vi "多从板对应参数.vi"(2 "从板个数":dbl=1.0) -> (0 "输出数组":string[](array[string]))   [LabVIEW 2013]
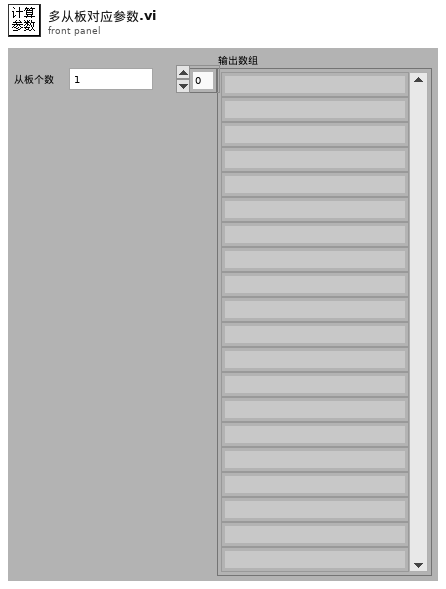
[diagram p1: front panel]
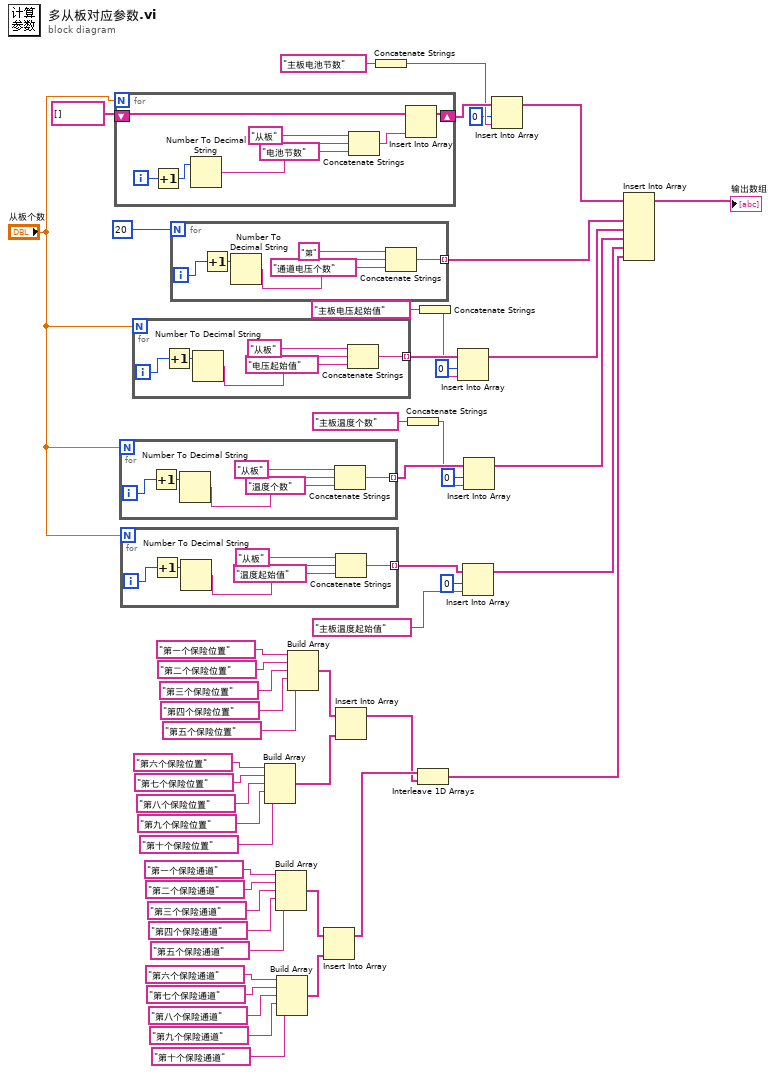
[diagram p0: block diagram]
diagram:
  n1 = for {
    N: "从板个数" -> [_]
    shift-right: [w56] -> w45
    shift-left: string[] [] -> [w55]
    i -> [w54]
    n2 = Increment(x=w54) -> (x+1=w52:i32)
    n3 = Number To Decimal String(number=w52) -> (decimal integer string=w58:string)  [unwired: 1 out]
    n4 = Concatenate Strings("从板" ("字符串"), w58, "电池节数" ("字符串")) -> (w53:string)
    n5 = Insert Into Array(array=w55, new element=w53) -> (w56:string[])  [unwired: 1 in]
  }
  n6 = for {
    N: "从板个数" -> [_]
    tunnel: [w60] -> w41 mode=indexing
    i -> [w65]
    n7 = Increment(x=w65) -> (x+1=w64:i32)
    n8 = Number To Decimal String(number=w64) -> (decimal integer string=w62:string)  [unwired: 1 out]
    n9 = Concatenate Strings("从板" ("字符串"), w62, "温度个数" ("字符串")) -> (w60:string)
  }
  n10 = for {
    N: "从板个数" -> [_]
    tunnel: [w66] -> w30 mode=indexing
    i -> [w71]
    n11 = Increment(x=w71) -> (x+1=w70:i32)
    n12 = Number To Decimal String(number=w70) -> (decimal integer string=w68:string)  [unwired: 1 out]
    n13 = Concatenate Strings("从板" ("字符串"), w68, "温度起始值" ("字符串")) -> (w66:string)
  }
  n14 = for {
    N: "从板个数" -> [_]
    tunnel: [w72] -> w37 mode=indexing
    i -> [w77]
    n15 = Increment(x=w77) -> (x+1=w76:i32)
    n16 = Number To Decimal String(number=w76) -> (decimal integer string=w74:string)  [unwired: 1 out]
    n17 = Concatenate Strings("从板" ("字符串"), w74, "电压起始值" ("字符串")) -> (w72:string)
  }
  n18 = for {
    N: 20 -> [_]
    tunnel: [w78] -> w48 mode=indexing
    i -> [w83]
    n19 = Increment(x=w83) -> (x+1=w82:i32)
    n20 = Number To Decimal String(number=w82) -> (decimal integer string=w80:string)  [unwired: 1 out]
    n21 = Concatenate Strings("第" ("字符串"), w80, "通道电压个数" ("字符串")) -> (w78:string)
  }
  n22 = Build Array("第六个保险位置" ("字符串"), "第七个保险位置" ("字符串"), "第八个保险位置" ("字符串"), "第九个保险位置" ("字符串"), "第十个保险位置" ("字符串")) -> (w16:string[])
  n23 = Build Array("第一个保险通道" ("字符串"), "第二个保险通道" ("字符串"), "第三个保险通道" ("字符串"), "第四个保险通道" ("字符串"), "第五个保险通道" ("字符串")) -> (w5:string[])
  n24 = Build Array("第六个保险通道" ("字符串"), "第七个保险通道" ("字符串"), "第八个保险通道" ("字符串"), "第九个保险通道" ("字符串"), "第十个保险通道" ("字符串")) -> (w4:string[])
  n25 = Build Array("第一个保险位置" ("字符串"), "第二个保险位置" ("字符串"), "第三个保险位置" ("字符串"), "第四个保险位置" ("字符串"), "第五个保险位置" ("字符串")) -> (w17:string[])
  n26 = Insert Into Array(array=w5, new element=w4) -> (w3:string[])  [unwired: 1 in]
  n27 = Insert Into Array(array=w17, new element=w16) -> (w2:string[])  [unwired: 1 in]
  n28 = Concatenate Strings("主板电池节数" ("字符串")) -> (w43:string)
  n29 = Concatenate Strings("主板温度个数" ("字符串")) -> (w39:string)
  n30 = Interleave 1D Arrays(w3, w2) -> (w1:string[])
  n31 = Concatenate Strings("主板电压起始值" ("字符串")) -> (w35:string)
  n32 = Insert Into Array(array=w37, index=0 ("索引"), new element=w35) -> (w33:string[])
  n33 = Insert Into Array(array=w30, index=0 ("索引"), new element="主板温度起始值" ("字符串")) -> (w29:string[])
  n34 = Insert Into Array(array=w41, index=0 ("索引"), new element=w39) -> (w32:string[])
  n35 = Insert Into Array(array=w45, index=0 ("索引"), new element=w43) -> (w46:string[])
  n36 = Insert Into Array(array=w46, new element #1=w48, new element #2=w33, new element #3=w32, new element #4=w29, new element #5=w1) -> (→"输出数组":string[])  [unwired: 1 in]
